vi "Main Algo Main Stream.vi"() -> ()   [LabVIEW 2015]
uses:
  Stream/Controls/RT Status Refs.ctl
  Stream/Controls/RT Streamer Queue element.ctl
  Stream/Controls/RT Streamer State.ctl
  Stream/LP Globals.vi
panel:
  in  "AutoBalance":bool
  in  "Set":bool
  in  "StatusRefs":T1
  out "output cluster":T2
  in  "AlgoRate":u8=10
  out "FrameRate":dbl
  out "Image Dst Out":T3(plugin-control)
  out "MaxY":u32
  out "MaxX":u32
  out "MaxB":u32
  out "MaxA":u32
  out "HorCenter":u16
  out "VerCenter":u32
  out "Algo Time":u32
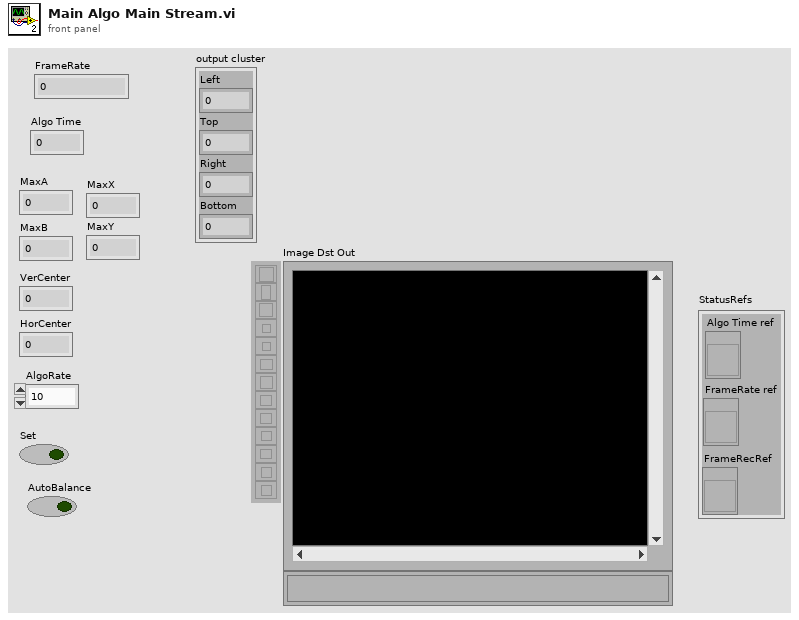
[diagram p1: front panel]
types:
  T1 = typedef "RT Status Refs.ctl" = cluster{"Algo Time ref":refnum<vi>, "FrameRate ref":refnum<vi>, "FrameRecRef":refnum<vi>}
  T2 = cluster{"Left":i32, "Top":i32, "Right":i32, "Bottom":i32}
  T3 = typedef "IMAQ Image.ctl" = refnum<image>
  T4 = typedef "RT Streamer Queue element.ctl" = cluster{"CMD":T5, "Data":variant}
  T5 = typedef "RT Streamer State.ctl" = enum16{"Init", "Idle", "Stream", "Listen", "SetRefrashRate", "SendCmdAck", "SendCmdDone", "SendSysState", "StartRecord", "Error"}
  T6 = typedef "Image Type" = u32
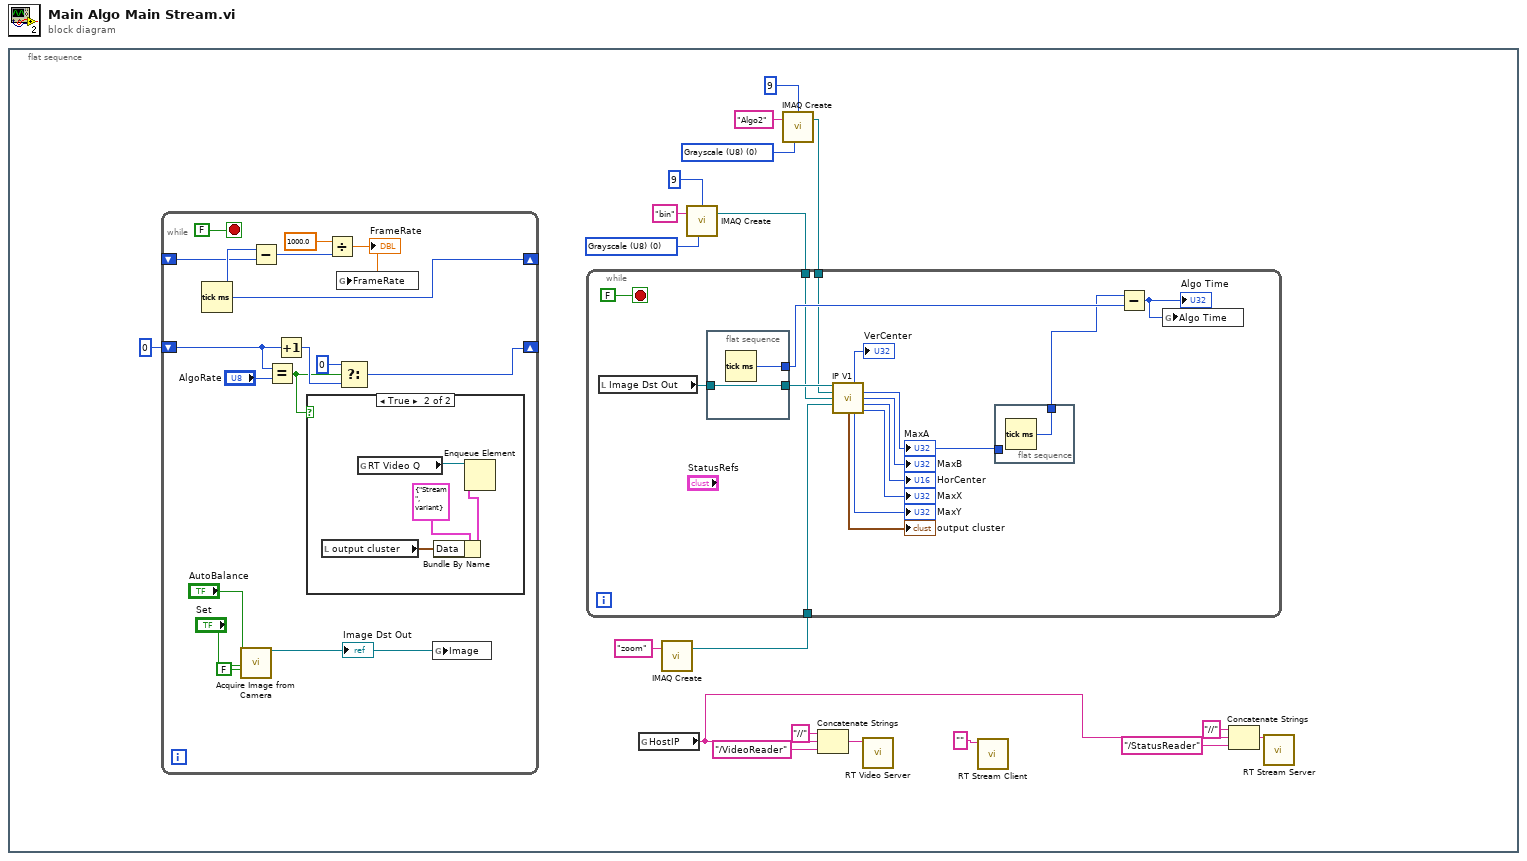
[diagram p0: block diagram]
diagram:
  n1 = flat-sequence {
    frame #0 {
      w11 = T6 0 items=["Grayscale (U8)", "Grayscale (I16)", "Grayscale (SGL)", "Complex (CSG)", "RGB (U32)", "HSL (U32)", "RGB (U64)", "Grayscale (U16)"] ("Image Type")
      w15 = T6 0 items=["Grayscale (U8)", "Grayscale (I16)", "Grayscale (SGL)", "Complex (CSG)", "RGB (U32)", "HSL (U32)", "RGB (U64)", "Grayscale (U16)"] ("Image Type")
      n2 = while {
        shift-right: [w52] -> _
        shift-left: _ -> [w51]
        shift-right: [w47] -> _
        shift-left: u8 0 -> [w49]
        stop <- FALSE stop-if-true
        n3 = Tick Count (ms)() -> (millisecond timer value=w52:u32)
        n4 = call "Acquire Image from Camera.vi"("AutoBalance"="AutoBalance", "Set"="Set", "Stop (F)"=FALSE) -> ("Image Out"=w42:T3)  [unwired: 22 in, 2 out]
        "Image Dst Out" <- w42
        n5 = Subtract(x=w52, y=w51) -> (x-y=w50:u32)
        n6 = Equal?(x=w49, y="AlgoRate") -> (x = y?=w45:bool)
        n7 = Increment(x=w49) -> (x+1=w48:u8)
        n8 = case shown="True" w45 {
          frame False {
          }
          frame True {
            n9 = local read "output cluster"() -> (w55:T2)
            n10 = global read "LP Globals.vi" "RT Video Q"() -> (w58:refnum<queue>)
            n11 = Bundle By Name(cluster=T4 {"CMD"=enum."Stream", "Data"=variant} ("element"), "Data"=w55) -> (w56:T4)
            n12 = Enqueue Element(queue=w58, element=w56) -> ()  [unwired: 2 in, 3 out]
          }
        }
        n13 = Divide(x=1000.0, y=w50) -> (x/y=w41:dbl)
        "FrameRate" <- w41
        n14 = global write "LP Globals.vi" "FrameRate"(w41) -> ()
        n15 = Select(t=u8 0, s=w45, f=w48) -> (s? t:f=w47:u8)
        n16 = global write "LP Globals.vi" "Image"(w42) -> ()
      }
      n17 = global read "LP Globals.vi" "HostIP"() -> (w3:string)
      n18 = call "IMAQ Create"("Image Name"="zoom") -> ("New Image"=w1:T3)  [unwired: 3 in, 2 out]
      n19 = call "IMAQ Create"("Border Size"=9, "Image Name"="bin", "Image Type"=w11) -> ("New Image"=w10:T3)  [unwired: 2 in, 1 out]
      n20 = call "IMAQ Create"("Border Size"=9, "Image Name"="Algo2", "Image Type"=w15) -> ("New Image"=w13:T3)  [unwired: 2 in, 1 out]
      n21 = while {
        tunnel: w13 -> [w24]
        tunnel: w10 -> [w23]
        tunnel: w1 -> [w20]
        stop <- FALSE stop-if-true
        n22 = local read "Image Dst Out"() -> (w25:T3)
        n23 = flat-sequence {
          tunnel: [w38] -> w29
          tunnel: w25 -> [w37]
          tunnel: [w37] -> w26
          frame #0 {
            n24 = Tick Count (ms)() -> (millisecond timer value=w38:u32)
          }
        }
        n25 = call "IP V1.vi"("Image In"=w26, "Image Dst"=w24, "BinImage"=w23, "Zoom Image"=w20) -> ("VerCenter"=→"VerCenter":u32, "MaxA"=w22:u32, "MaxB"=→"MaxB":u32, "HorCenter"=→"HorCenter":u16, "output cluster"=→"output cluster":T2, "MaxY"=→"MaxY":u32, "MaxX"=→"MaxX":u32)  [unwired: 4 in, 1 out]
        "MaxA" <- w22
        n26 = flat-sequence {
          tunnel: [w36] -> w27
          tunnel: w22 -> [_]
          frame #0 {
            n27 = Tick Count (ms)() -> (millisecond timer value=w36:u32)
          }
        }
        n28 = Subtract(x=w27, y=w29) -> (x-y=w21:u32)
        "Algo Time" <- w21
        n29 = global write "LP Globals.vi" "Algo Time"(w21) -> ()
      }
      n30 = Concatenate Strings("//" ("string"), w3, "/VideoReader" ("reader url")) -> (w16:string)
      n31 = call "RT Video Server.vi"("reader url"=w16) -> ()  [unwired: 11 in]
      n32 = call "RT Stream Client.vi"("Writer url"="") -> ()  [unwired: 11 in]
      n33 = Concatenate Strings("//" ("string"), w3, "/StatusReader" ("reader url")) -> (w5:string)
      n34 = call "RT Stream Server.vi"("reader url"=w5) -> ()  [unwired: 11 in]
    }
  }
